vi "Raw data Reader  AD4212C(SubVI).vi"(6 "error in (no error)":errorcluster, 9 "VISA Refnum in":refnum<visa-resource-name>) -> (0 "error out":errorcluster, 1 "Peso":dbl, 2 "read buffer":string, 3 "VISA reference":refnum<visa-resource-name>)   [LabVIEW 2014, in "AD4212C.lvlib"]
uses:
  AD4212C.lvlib
  Control 1.ctl
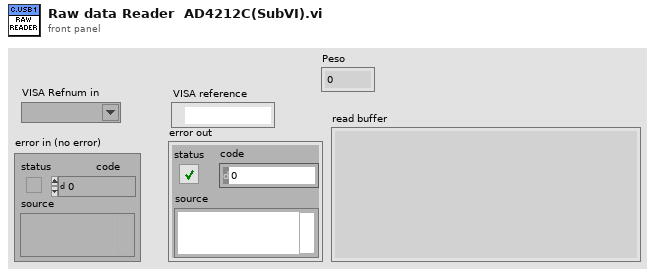
[diagram p1: front panel]
types:
  T1 = typedef "Control 1.ctl" = enum16{"IDLE", "Detect 01"}
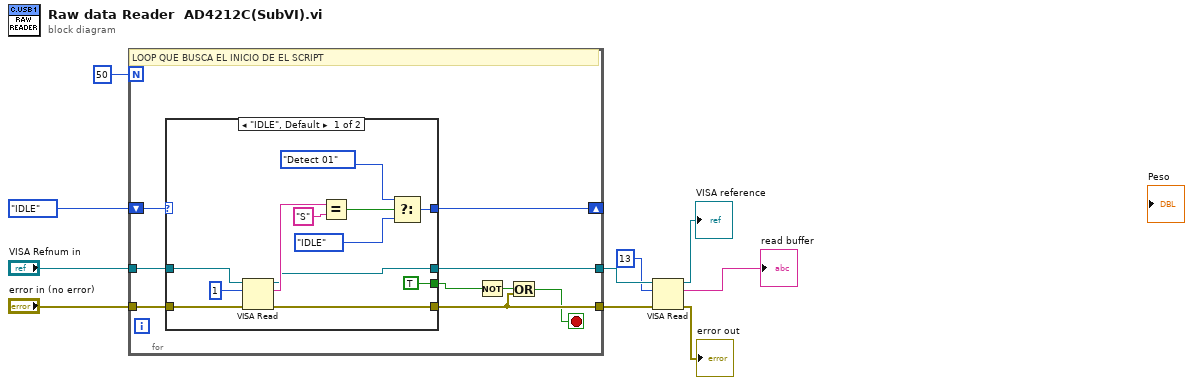
[diagram p0: block diagram]
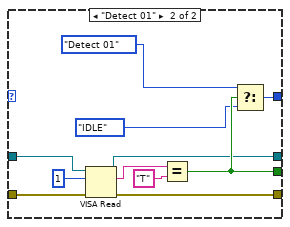
[diagram p2: hidden frame]
diagram:
  n1 = for {
    N: 50 -> [_]
    tunnel: "VISA Refnum in" -> [w19]
    tunnel: "error in (no error)" -> [w18]
    shift-right: [w16] -> _
    shift-left: enum16{"IDLE", "Detect 01"}."IDLE" ("Enum") -> [w17]
    tunnel: [w15] -> w7
    tunnel: [w12] -> w6
    stop <- w11 stop-if-true
    # "LOOP QUE BUSCA EL INICIO DE EL SCRIPT"
    n2 = case shown="\"IDLE\", Default" w17 {
      tunnel: w19 -> [w24 w37]
      tunnel: w18 -> [w31 w38]
      tunnel: [w28 w40] -> w16
      tunnel: [TRUE w35] -> w13
      tunnel: [w20 w32] -> w15
      tunnel: [w23 w36] -> w12
      frame "IDLE", Default {
        n3 = VISA Read(VISA resource name=w24, byte count=u32 1, error in (no error)=w31) -> (VISA resource name out=w20:refnum<visa-resource-name>, read buffer=w26:string, error out=w23:errorcluster)  [unwired: 1 out]
        n4 = Equal?(x=w26, y="S") -> (x = y?=w27:bool)
        n5 = Select(t=enum16{"IDLE", "Detect 01"}."Detect 01" ("Enum"), s=w27, f=enum16{"IDLE", "Detect 01"}."IDLE" ("Enum")) -> (s? t:f=w28:enum16{"IDLE", "Detect 01"})
      }
      frame "Detect 01" {
        n6 = VISA Read(VISA resource name=w37, byte count=u32 1, error in (no error)=w38) -> (VISA resource name out=w32:refnum<visa-resource-name>, read buffer=w39:string, error out=w36:errorcluster)  [unwired: 1 out]
        n7 = Equal?(x=w39, y="T") -> (x = y?=w35:bool)
        n8 = Select(t=Control_1."Detect 01" ("Enum"), s=w35, f=Control_1."IDLE" ("Enum")) -> (s? t:f=w40:T1)
      }
    }
    n9 = Not(x=w13) -> (.not. x?=w14:bool)
    n10 = Or(x=w14, y=w12) -> (x .or. y?=w11:bool)
  }
  n11 = VISA Read(VISA resource name=w7, byte count=u32 13, error in (no error)=w6) -> (VISA resource name out=→"VISA reference":refnum<visa-resource-name>, read buffer=→"read buffer":string, error out=→"error out":errorcluster)  [unwired: 1 out]
